vi "NI VeriStand - Set Item GUID.vi"(6 "Refresh System Explorer Tree? (F)":bool, 8 "error in (no error)":errorcluster, 9 "GUID":string, 11 "Item Ref in":T1 format="%.0x") -> (0 "error out":errorcluster, 3 "Item Ref out":T1 format="%.0x")   [LabVIEW 2020, in "Custom Device Offline API.lvlib"]
uses:
  <vilib>/NI VeriStand/Custom Device Offline API/Custom Device Offline API.lvlib
  <vilib>/NI VeriStand/Custom Device API/Custom Device Item Ref.ctl
  NationalInstruments.VeriStand.SystemDefinitionAPI
  <vilib>/NI VeriStand/Custom Device API/Custom Device API.lvlib
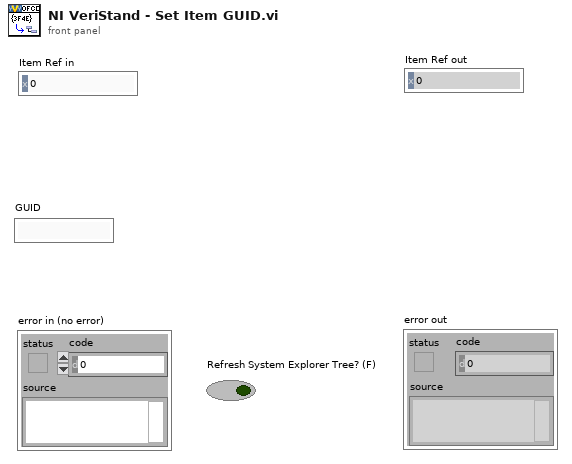
[diagram p1: front panel]
types:
  T1 = typedef "Custom Device API.lvlib/Custom Device Item Ref.ctl" = u64
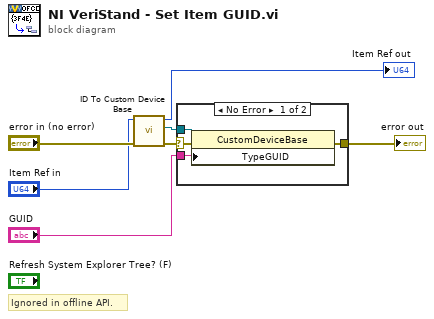
[diagram p0: block diagram]
diagram:
  # "Ignored in offline API."
  n1 = call <vilib>:"ID To Custom Device Base.vi"("error in (no error)"="error in (no error)", "ID in"="Item Ref in") -> ("error out"=w5:errorcluster, "BaseNode"=w4:refnum<k24>, "ID out"=→"Item Ref out":u64)  [unwired: 7 in]
  n2 = case shown="No Error" w5 {
    selector: w5 -> [w10 w12]
    tunnel: w4 -> [w11 _]
    tunnel: "GUID" -> [w9 _]
    tunnel: [w8 w12] -> w2
    frame No Error {
      n3 = property class="CustomDeviceBase"(reference=w11, error in=w10, "TypeGUID"=w9) -> (error out=w8:errorcluster)  [unwired: 1 out]
    }
    frame Error {
    }
  }
  "error out" <- w2
